vi "Mass Edit Icon.vi"() -> ()   [LabVIEW 2020]
uses:
  <userlib>/_OpenG.lib/file/file.llb/openg_file.lvlib
panel:
  in  "Glyph Root":path
  out "file paths":path[](array[path])
  out "error out":errorcluster
  out "N":i32
  out "i":i32
  in  "error in (no error)":errorcluster
  in  "CTL Root":path
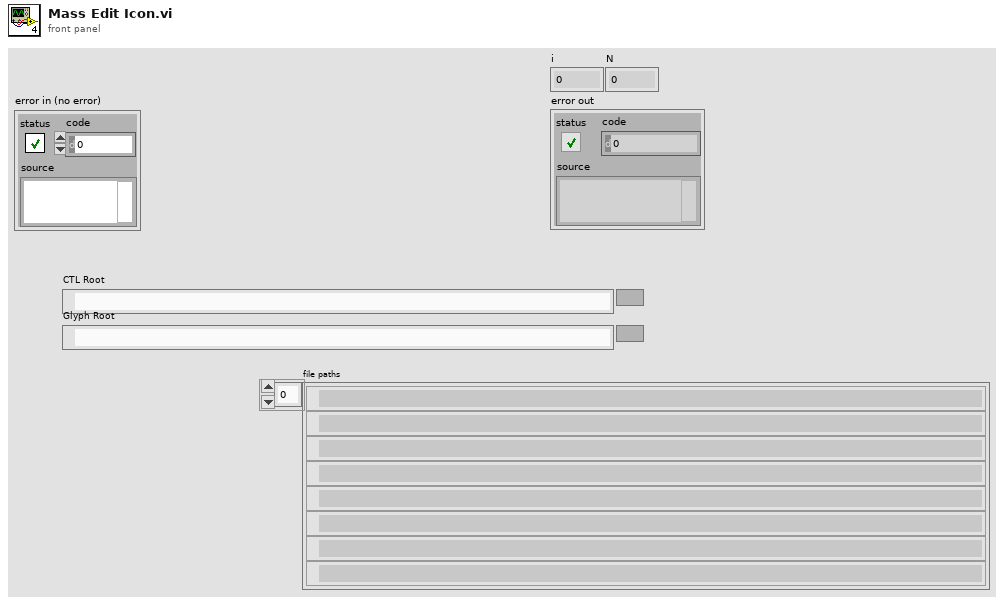
[diagram p1: front panel]
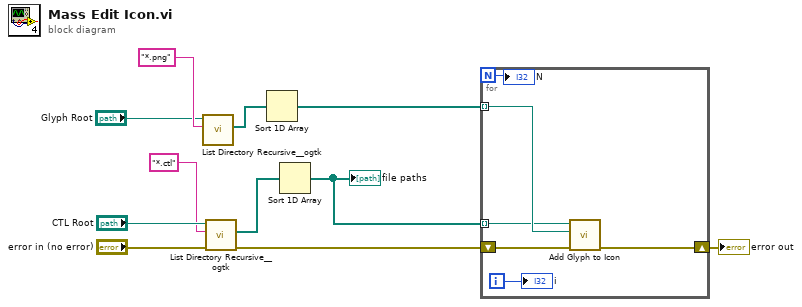
[diagram p0: block diagram]
diagram:
  n1 = call <userlib>:"List Directory Recursive__ogtk.vi"("pattern"="*.png", "Path"="Glyph Root") -> ("file paths"=w4:path[])  [unwired: 6 in, 3 out]
  n2 = call <userlib>:"List Directory Recursive__ogtk.vi"("error in (no error)"="error in (no error)", "pattern"="*.ctl", "Path"="CTL Root") -> ("error out"=w8:errorcluster, "file paths"=w3:path[])  [unwired: 5 in, 2 out]
  n3 = Sort 1D Array(array=w4) -> (sorted array=w1:path[])
  n4 = Sort 1D Array(array=w3) -> (sorted array=w2:path[])
  "file paths" <- w2
  n5 = for {
    N -> [w16]
    tunnel: w2 -> [w12] mode=indexing
    shift-right: [w14] -> w7
    shift-left: w8 -> [w15]
    tunnel: w1 -> [w13] mode=indexing
    i -> [w17]
    n6 = call "Add Glyph to Icon.vi"("error in (no error)"=w15, "Glyph Path"=w13, "Control Path"=w12) -> ("error out"=w14:errorcluster)  [unwired: 8 in]
    "i" <- w17
    "N" <- w16
  }
  "error out" <- w7
